vi "Get Thread ID Pool.vi"(11 "Transceiver Thread in":refnum<class "Plugin Thread.lvclass">) -> (2 "Thread ID Pool":refnum<class "ID Pool.lvclass">, 3 "Transceiver Thread out":refnum<class "Plugin Thread.lvclass">)   [LabVIEW 2017, in "DSF Core.lvlib" / "Plugin Thread.lvclass"]
uses:
  Plugin Thread.lvclass
  Thread Pool/ID Pool.lvclass
  Plugin Thread.lvclass/Plugin Thread.ctl
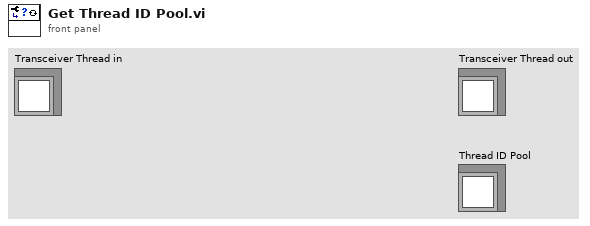
[diagram p1: front panel]
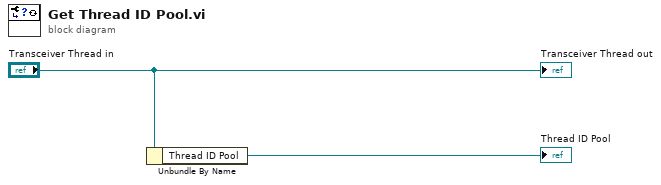
[diagram p0: block diagram]
diagram:
  n1 = Unbundle By Name("Transceiver Thread in") -> ("Thread ID Pool"=→"Thread ID Pool":refnum<class "ID Pool.lvclass">)
  "Transceiver Thread out" <- "Transceiver Thread in"
